vi "Broadcast Metadata.vi"(8 "error in (no error)":errorcluster, 11 "Log Record in":refnum<class "Log Record.lvclass">) -> (0 "error out":errorcluster, 3 "Log Record out":refnum<class "Log Record.lvclass">)   [LabVIEW 2021, in "Log Record.lvclass"]
uses:
  Log Record.lvclass
  C:/Program Files/National Instruments/LabVIEW 2021/vi.lib/ActorFramework/Actor/Actor.lvclass
  NHMFL_Core/Libraries/File/Metadata/Metadata.lvclass
  Worker/Worker Messages/Add Metadata Msg/Add Metadata Msg.lvclass
  C:/Program Files/National Instruments/LabVIEW 2021/vi.lib/ActorFramework/Message/Message.lvclass
  <vilib>/ActorFramework/Actor/Actor.lvclass/Actor.ctl
  Log Record.lvclass/Log Record.ctl
  Template Module Messages/Message Nested Object Msg/Message Nested Object Msg.lvclass/Message Nested Object Msg.ctl
  <vilib>/ActorFramework/Message Enqueuer/Message Enqueuer.lvclass/Message Enqueuer.ctl
  <vilib>/ActorFramework/Message Enqueuer/Enqueue.vi
  Template Module Messages/Message Nested Object Msg/Message Nested Object Msg.lvclass
  <vilib>/ActorFramework/Message Priority Queue/Priority Enqueue.vi
  <vilib>/ActorFramework/Actor/Actor.lvclass
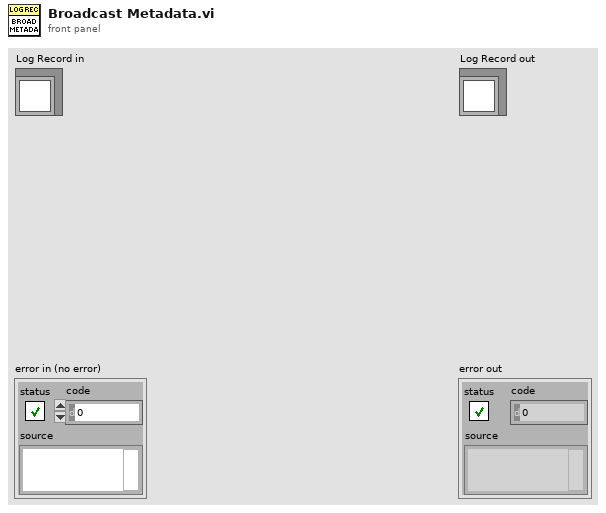
[diagram p1: front panel]
types:
  T1 = typedef "Log Record Configuration.ctl" = cluster{"OSF node  ID":string, "Conection timeout":dbl, "Station":string, "Log server ":string, "Upload to OSF":bool, "Append to lab book":bool, "Filing modules":string[]}
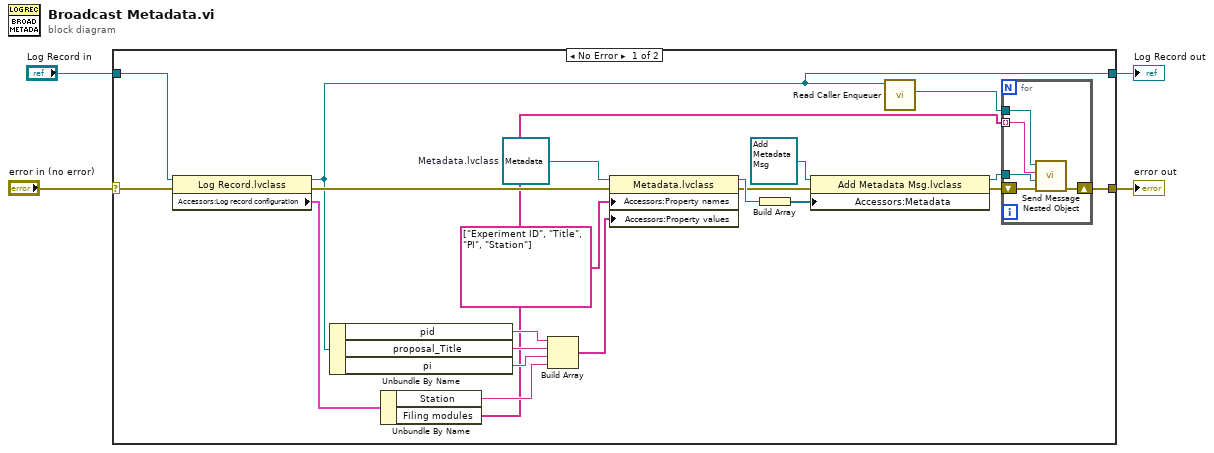
[diagram p0: block diagram]
diagram:
  n1 = case shown="No Error" "error in (no error)" {
    selector: "error in (no error)" -> [w25 w32]
    tunnel: [w6 w32] -> w3
    tunnel: [w13 w31] -> w1
    tunnel: "Log Record in" -> [w24 w31]
    frame No Error {
      w22 = refnum<class "Metadata.lvclass"> refnum  # Metadata.lvclass
      n2 = property class="Log Record.lvclass"(reference=w24, error in=w25) -> (reference out=w13:refnum<class "Log Record.lvclass">, error out=w21:errorcluster, "Accessors:Log record configuration"=w23:T1)
      n3 = Unbundle By Name(w13) -> ("pid"=w19:string, "proposal_Title"=w18:string, "pi"=w17:string)
      n4 = Unbundle By Name(w23) -> ("Station"=w16:string, "Filing modules"=w14:string[])
      n5 = Build Array(w19, w18, w17, w16) -> (w15:string[])
      n6 = property class="Metadata.lvclass"(reference=w22, error in=w21, "Accessors:Property names"=string[] ["Experiment ID", "Title", "PI", "Station"], "Accessors:Property values"=w15) -> (reference out=w10:refnum<class "Metadata.lvclass">, error out=w8:errorcluster)
      n7 = Build Array(w10) -> (w9:refnum<class "Metadata.lvclass">[])
      n8 = property class="Add Metadata Msg.lvclass"(reference=refnum<class "Add Metadata Msg.lvclass"> refnum ("Add Metadata Msg.lvclass"), error in=w8, "Accessors:Metadata"=w9) -> (reference out=w5:refnum<class "Add Metadata Msg.lvclass">, error out=w7:errorcluster)
      n9 = call <vilib>:"Read Caller Enqueuer.vi"("Actor"=w13) -> ("Caller Enqueuer"=w12:refnum<class "Message Enqueuer.lvclass">)  [unwired: 10 in]
      n10 = for {
        tunnel: w14 -> [w29] mode=indexing
        tunnel: w12 -> [w30]
        shift-right: [w27] -> w6
        shift-left: w7 -> [w28]
        tunnel: w5 -> [w26]
        n11 = call "Send Message Nested Object.vi"("error in (no error)"=w28, "Message"=w26, "Name"=w29, "Message Enqueuer"=w30) -> ("error out"=w27:errorcluster)  [unwired: 6 in, 1 out]
      }
    }
    frame Error {
    }
  }
  "error out" <- w3
  "Log Record out" <- w1
